vi "Interpolate.vi"(1 "Last Scan":dbl[](array[numeric]) format="%.2f", 2 "First Scan":dbl[](array[numeric]) format="%.2f", 3 "Length":i32) -> (0 "Ramp Pattern":dbl[][](array[numeric]) format="%.2f")   [LabVIEW 2013]
uses:
  <vilib>/Analysis/1siggen.llb/Ramp Pattern by Samples.vi
  <vilib>/Analysis/NI_AALBase.lvlib
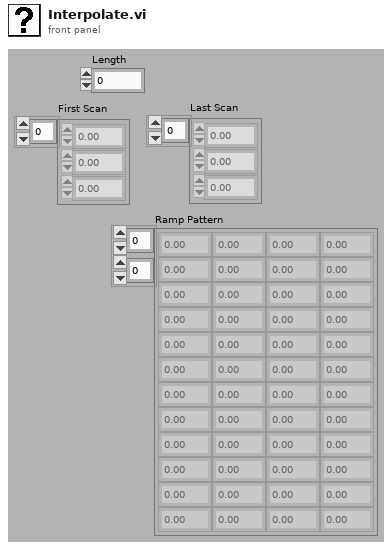
[diagram p1: front panel]
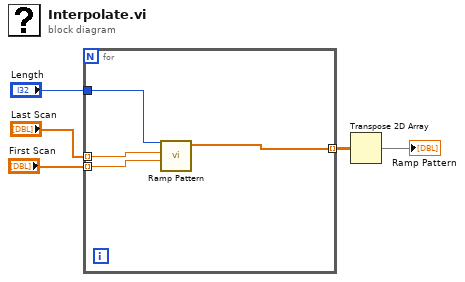
[diagram p0: block diagram]
diagram:
  n1 = for {
    tunnel: "First Scan" -> [w9] mode=indexing
    tunnel: "Last Scan" -> [w8] mode=indexing
    tunnel: "Length" -> [w7]
    tunnel: [w6] -> w2 mode=indexing
    n2 = call-poly <vilib>:"Ramp Pattern.vi"("start"=w9, "end"=w8, "samples"=w7) -> ("Ramp Pattern"=w6:dbl[])  [unwired: 7 in, 1 out]
  }
  n3 = Transpose 2D Array(2D array=w2) -> (transposed array=→"Ramp Pattern":dbl[][])
